vi "LPF.vi"(6 "initialize":bool, 9 "low cutoff freq: fl":dbl=10.0, 10 "sampling freq: fs":dbl=1000.0, 11 "Planned Tension in":dbl[](array[numeric])) -> (3 "Planned Tension out":dbl[](array[numeric]))   [LabVIEW 2016]
uses:
  <vilib>/ptbypt/NI_PtbyPt.lvlib
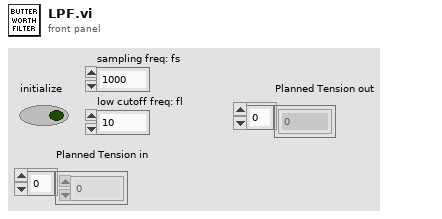
[diagram p1: front panel]
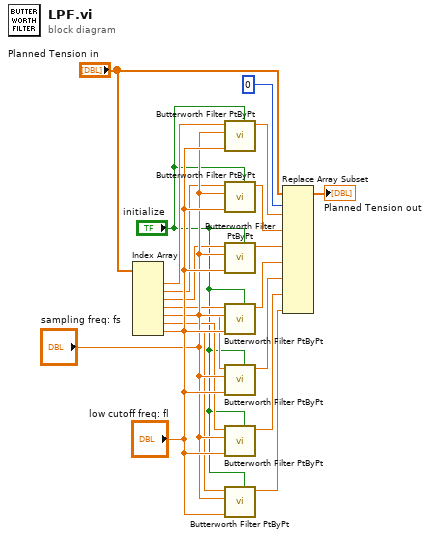
[diagram p0: block diagram]
diagram:
  n1 = Index Array(array="Planned Tension in") -> (element #1=w2:dbl, element #2=w3:dbl, element #3=w4:dbl, element #4=w5:dbl, element #5=w6:dbl, element #6=w7:dbl, element #7=w8:dbl)  [unwired: 7 in]
  n2 = call <vilib>:"Butterworth Filter PtByPt.vi"("initialize"="initialize", "low cutoff freq: fl"="low cutoff freq: fl", "sampling freq: fs"="sampling freq: fs", "x"=w2) -> ("Filtered x"=w13:dbl)  [unwired: 5 in, 1 out]
  n3 = call <vilib>:"Butterworth Filter PtByPt.vi"("initialize"="initialize", "low cutoff freq: fl"="low cutoff freq: fl", "sampling freq: fs"="sampling freq: fs", "x"=w3) -> ("Filtered x"=w14:dbl)  [unwired: 5 in, 1 out]
  n4 = call <vilib>:"Butterworth Filter PtByPt.vi"("initialize"="initialize", "low cutoff freq: fl"="low cutoff freq: fl", "sampling freq: fs"="sampling freq: fs", "x"=w4) -> ("Filtered x"=w15:dbl)  [unwired: 5 in, 1 out]
  n5 = call <vilib>:"Butterworth Filter PtByPt.vi"("initialize"="initialize", "low cutoff freq: fl"="low cutoff freq: fl", "sampling freq: fs"="sampling freq: fs", "x"=w5) -> ("Filtered x"=w16:dbl)  [unwired: 5 in, 1 out]
  n6 = call <vilib>:"Butterworth Filter PtByPt.vi"("initialize"="initialize", "low cutoff freq: fl"="low cutoff freq: fl", "sampling freq: fs"="sampling freq: fs", "x"=w6) -> ("Filtered x"=w17:dbl)  [unwired: 5 in, 1 out]
  n7 = call <vilib>:"Butterworth Filter PtByPt.vi"("initialize"="initialize", "low cutoff freq: fl"="low cutoff freq: fl", "sampling freq: fs"="sampling freq: fs", "x"=w7) -> ("Filtered x"=w18:dbl)  [unwired: 5 in, 1 out]
  n8 = call <vilib>:"Butterworth Filter PtByPt.vi"("initialize"="initialize", "low cutoff freq: fl"="low cutoff freq: fl", "sampling freq: fs"="sampling freq: fs", "x"=w8) -> ("Filtered x"=w19:dbl)  [unwired: 5 in, 1 out]
  n9 = Replace Array Subset(array="Planned Tension in", new element #1=w13, index #1=0 ("index"), new element #2=w14, new element #3=w15, new element #4=w16, new element #5=w17, new element #6=w18, new element #7=w19) -> (→"Planned Tension out":dbl[])  [unwired: 6 in]
